vi "iterate_folder_name.vi"(11 "Folder In":path) -> (3 "Folder Out":path)   [LabVIEW 2015]
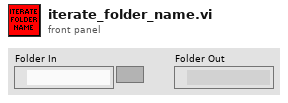
[diagram p1: front panel]
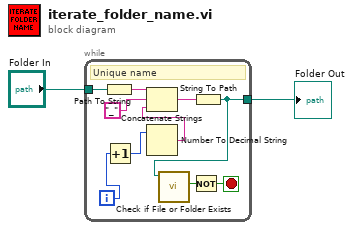
[diagram p0: block diagram]
diagram:
  n1 = while {
    tunnel: "Folder In" -> [w10]
    tunnel: [w7] -> w1
    i -> [w3]
    stop <- w9 stop-if-true
    # "Unique name"
    n2 = Path To String(path=w10) -> (string=w11:string)
    n3 = Increment(x=w3) -> (x+1=w4:i32)
    n4 = Number To Decimal String(number=w4) -> (decimal integer string=w6:string)  [unwired: 1 in]
    n5 = Concatenate Strings(w11, "_", w6) -> (w5:string)
    n6 = String To Path(string=w5) -> (path=w7:path)
    n7 = call <vilib>:"Check if File or Folder Exists.vi"("path"=w7) -> ("file or folder exists?"=w8:bool)  [unwired: 8 in, 2 out]
    n8 = Not(x=w8) -> (.not. x?=w9:bool)
  }
  "Folder Out" <- w1
